vi "PortControl.vi"(1 "Function":enum16{"OpenPort", "ClosePort"}(ring), 5 "baud rate (9600)":u32=9600 caption="波特率(9600)", 7 "data bits (8)":u16=8 caption="数据比特(8)" min=5 max=8 step=1, 9 "stop bits (10: 1 bit)":u16(ring)=10 caption="停止位（10: 1位）" items=["1.0"=10, "1.5"=15, "2.0"=20], 11 "parity (0:none)":enum16{"None", "Odd", "Even", "Mark", "Space"}(ring) caption="奇偶（0:无）") -> (4 "return":bool)   [LabVIEW 2013]
uses:
  <vilib>/Instr/_visa.llb/VISA Configure Serial Port (Instr).vi
panel:
  in  "PortName":string
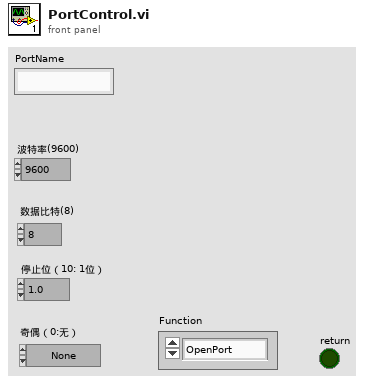
[diagram p1: front panel]
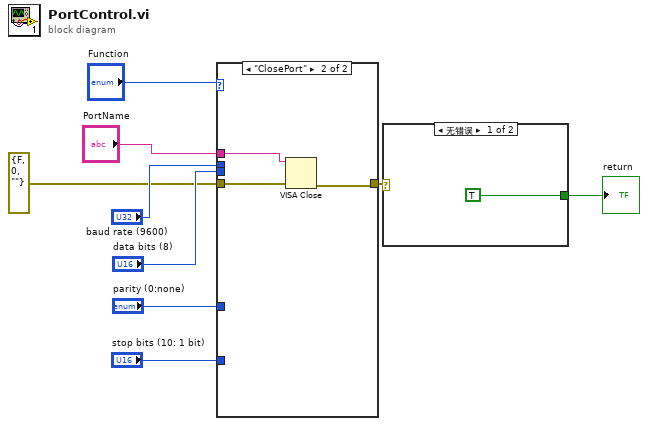
[diagram p0: block diagram]
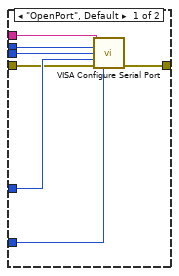
[diagram p2: hidden frame]
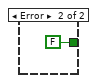
[diagram p3: hidden frame]
diagram:
  n1 = case shown="\"ClosePort\"" "Function" {
    tunnel: "baud rate (9600)" -> [w16 _]
    tunnel: "data bits (8)" -> [w15 _]
    tunnel: "parity (0:none)" -> [w14 _]
    tunnel: "stop bits (10: 1 bit)" -> [w13 _]
    tunnel: errorcluster {"status"=FALSE, "code"=0, "source"=""} ("error in (no error)") -> [w12 w18]
    tunnel: "PortName" -> [w11 w17]
    tunnel: [w10 w19] -> w3
    frame "OpenPort", Default {
      n2 = call-poly "VISA Configure Serial Port"("VISA resource name"=w11, "baud rate (9600)"=w16, "data bits (8)"=w15, "parity (0:none)"=w14, "error in (no error)"=w12, "stop bits (10: 1 bit)"=w13) -> ("error out"=w10:errorcluster)  [unwired: 8 in, 1 out]
    }
    frame "ClosePort" {
      n3 = VISA Close(VISA resource name=w17, error in (no error)=w18) -> (error out=w19:errorcluster)
    }
  }
  n4 = case shown="无错误" w3 {
    tunnel: [TRUE ("status") FALSE ("status")] -> w2
    frame No Error {
    }
    frame Error {
    }
  }
  "return" <- w2
